vi "Time.vi"(8 "error in (no error)":errorcluster, 10 "Control In":T1, 11 "Crosshair Dispense in":refnum<class "Crosshair Dispense.lvclass">) -> (0 "error out":errorcluster, 1 "Timing Data":i32[](array[numeric]), 2 "Control Out":T1, 3 "Crosshair Dispense out":refnum<class "Crosshair Dispense.lvclass">)   [LabVIEW 2019, in "Crosshair Dispense.lvclass"]
uses:
  Crosshair Dispense.lvclass
  Controller/Controllers.ctl
  Controller/I-O/I-O.lvclass
  Controller/Dispenser/Dispenser.lvclass
  C:/Program Files (x86)/Aerotech/A3200/LabVIEW/2010/Bin/Aerotech.A3200.dll
  Program Files (x86)/Aerotech/A3200/LabVIEW/2010/Bin/Aerotech.A3200.dll
  Crosshair Dispense.lvclass/Crosshair Dispense.ctl
  Controller/Motion/A3200/A3200.lvclass
  Controller/Controller.lvclass
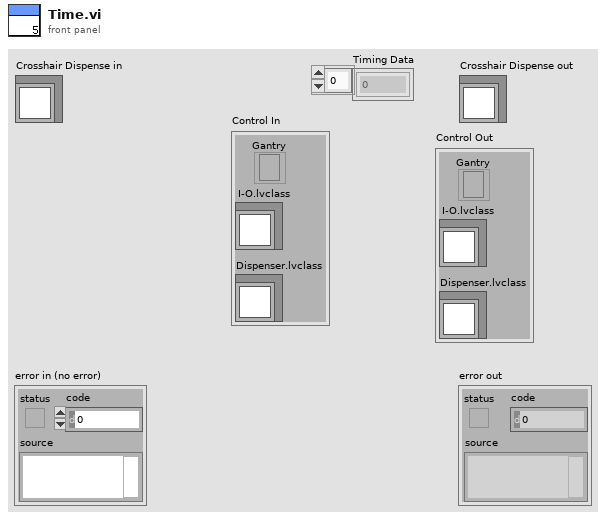
[diagram p1: front panel]
types:
  T1 = typedef "Controller.lvclass/Controllers.ctl" = cluster{"I-O.lvclass":refnum<class "I-O.lvclass">, "Dispenser.lvclass":refnum<class "Dispenser.lvclass">, "Gantry":refnum<k24>}
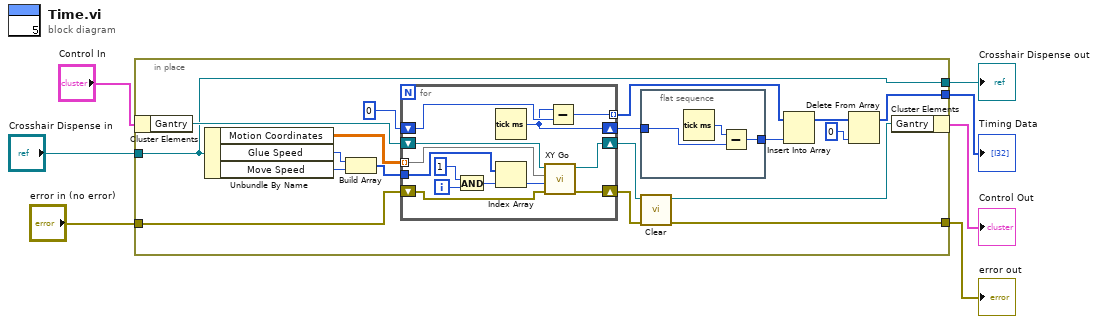
[diagram p0: block diagram]
diagram:
  n1 = in-place {
    in-place-border: "Crosshair Dispense in" -> [w8]
    in-place-border: [w15] -> w4
    in-place-border: "error in (no error)" -> [w11]
    in-place-border: [w9] -> w6
    in-place-border: [w8] -> w1
    n2 = in-place-cluster #1("Control In") -> ("Gantry"=w14:refnum<k24>)
    n3 = Unbundle By Name(w8) -> ("Motion Coordinates"=w16:dbl[][], "Glue Speed"=w18:i32, "Move Speed"=w17:i32)
    n4 = Build Array(w18, w17) -> (w19:i32[])
    n5 = for {
      shift-right: [w36] -> w20
      shift-left: u32 0 ("millisecond timer value") -> [w39]
      tunnel: [w38] -> w22 mode=indexing
      tunnel: w16 -> [w29] mode=indexing
      tunnel: w19 -> [w34]
      shift-right: [w32] -> w13
      shift-left: w14 -> [w33]
      shift-right: [w30] -> w10
      shift-left: w11 -> [w31]
      i -> [w40]
      n6 = And(x=1, y=w40) -> (x .and. y?=w37:i32)
      n7 = Tick Count (ms)() -> (millisecond timer value=w36:u32)
      n8 = Index Array(array=w34, index=w37) -> (element=w35:i32)
      n9 = call "XY Go.vi"("error in (no error)"=w31, "Speed"=w35, "XY"=w29, "Gantry In"=w33) -> ("error out"=w30:errorcluster, "Gantry Out"=w32:refnum<k24>)  [unwired: 6 in]
      n10 = Subtract(x=w36, y=w39) -> (x-y=w38:u32)
    }
    n11 = flat-sequence {
      tunnel: [w27] -> w23
      tunnel: w20 -> [w26]
      frame #0 {
        n12 = Tick Count (ms)() -> (millisecond timer value=w28:u32)
        n13 = Subtract(x=w28, y=w26) -> (x-y=w27:u32)
      }
    }
    n14 = call "Clear.vi"("error in (no error)"=w10, "Gantry In"=w13) -> ("error out"=w9:errorcluster, "Gantry Out"=w12:refnum<k24>)  [unwired: 8 in]
    n15 = Insert Into Array(array=w22, new element=w23) -> (w21:u32[])  [unwired: 1 in]
    n16 = Delete From Array(array=w21, index=0) -> (array with subset deleted=w15:u32[])  [unwired: 1 in, 1 out]
    n17 = in-place-cluster #1("Gantry"=w12) -> (→"Control Out":T1)
  }
  "error out" <- w6
  "Crosshair Dispense out" <- w1
  "Timing Data" <- w4
